vi "Write_TextFile.vi"(9 "Fecha":timestamp format="%^<%H:%M:%S>T", 11 "Producto":string) -> ()   [LabVIEW 2017]
doc: "Escribir en Text File."
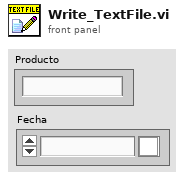
[diagram p1: front panel]
types:
  T1 = enum16{"open", "replace", "create", "open or create", "replace or create", "replace or create with confirmation"}
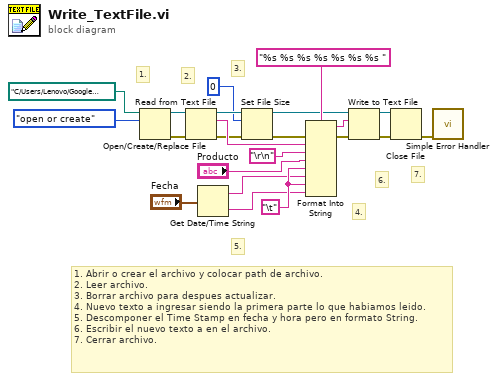
[diagram p0: block diagram]
diagram:
  w11 = "\t"
  # "1. Abrir o crear el archivo y colocar path de archivo.\n2. Leer archivo.\n3. Borrar archivo para despues actualizar.\n4. Nuevo texto a ingresar siendo la primera parte lo que habiamos leido.\n5. Descomponer el Time Stamp en fecha y hora pero en formato String.\n6. Escribir el nuevo texto a en el archivo.\n7. Cerrar archivo."
  # "7."
  # "6."
  # "5."
  # "4."
  # "3."
  # "2."
  # "1."
  n1 = Open/Create/Replace File(file path (use dialog)=path "C:/Users/Lenovo/Google Drive/Labview/Curso (FIME)/HW/Act. 3/HW. 3/Stuff/Historial.txt", operation (0:open)=T1."open or create") -> (refnum out=w14:refnum<file>, error out=w15:errorcluster)  [unwired: 4 in, 1 out]
  n2 = Read from Text File(file (use dialog)=w14, error in=w15) -> (refnum out=w9:refnum<file>, text=w13:string, error out=w10:errorcluster)  [unwired: 2 in, 1 out]
  n3 = Get Date/Time String(seconds (now)="Fecha") -> (date string=w2:string, time string=w1:string)  [unwired: 2 in]
  n4 = Set File Size(4:w10, 6:i64 0 ("size (in bytes)"), 7:w9) -> (0:w6:errorcluster, 3:w7:refnum<file>)
  n5 = Format Into String(format string="%s %s %s %s %s %s %s ", error in=w6, w13, "\r\n", "Producto", w11, w2, w11, w1) -> (resulting string=w18:string, error out=w17:errorcluster)  [unwired: 1 in]
  n6 = Write to Text File(file (use dialog)=w7, text=w18, error in=w17) -> (refnum out=w21:refnum<file>, error out=w20:errorcluster)  [unwired: 1 in, 1 out]
  n7 = Close File(refnum=w21, error in=w20) -> (error out=w19:errorcluster)  [unwired: 1 out]
  n8 = call <vilib>:"Simple Error Handler.vi"("error in (no error)"=w19) -> ()  [unwired: 4 in, 5 out]
